vi "generate sensorion data log header.vi"(5 "line ending (\"\", none)":string, 7 "delimiter (comma)":string=", ", 9 "index format (-%02d)":string="%02d", 10 "num sensors":i32, 11 "header format (%15s)":string="%15s") -> (1 "delimiter":string, 2 "sensor data header string":string, 3 "value format":string)   [LabVIEW 2021]
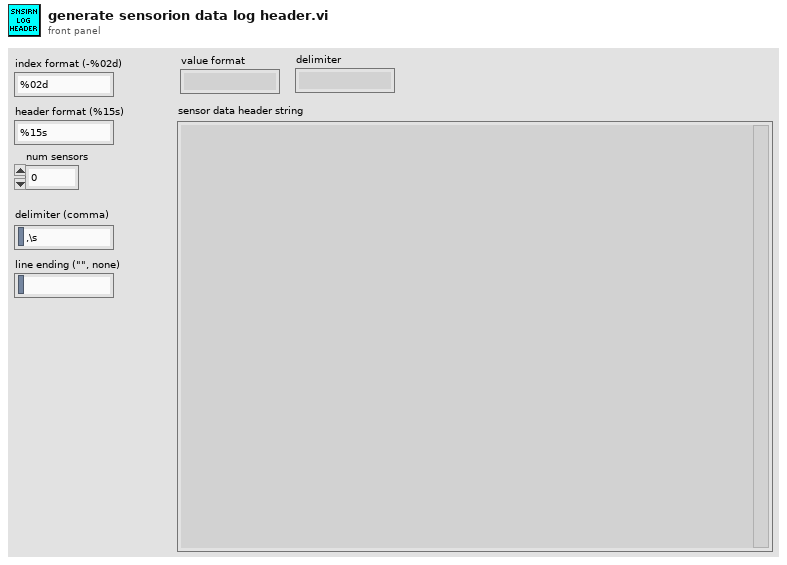
[diagram p1: front panel]
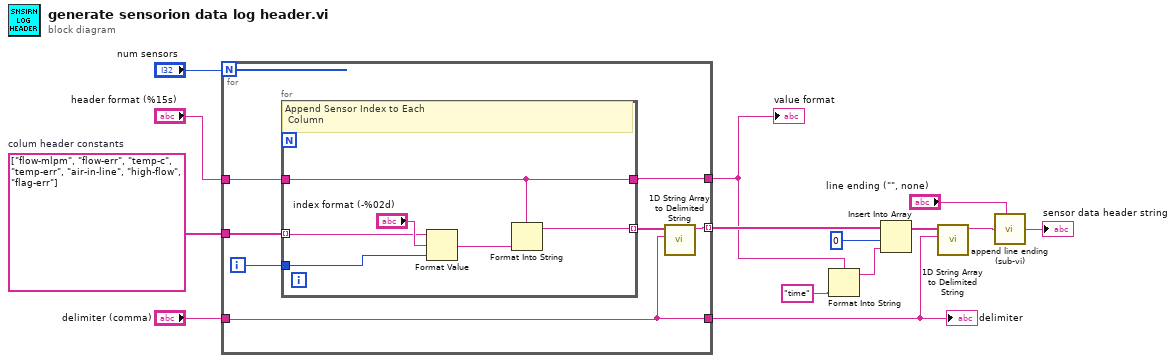
[diagram p0: block diagram]
diagram:
  w13 = string[] ["flow-mlpm", "flow-err", "temp-c", "temp-err", "air-in-line", "high-flow", "flag-err"]  # colum header constants
  n1 = for {
    N: "num sensors" -> [_]
    tunnel: w13 -> [w21]
    tunnel: "delimiter (comma)" -> [w18]
    tunnel: [w19] -> w9 mode=indexing
    tunnel: [w18] -> w11
    tunnel: "header format (%15s)" -> [w16]
    tunnel: [w15] -> w1
    i -> [w17]
    n2 = for {
      tunnel: w21 -> [w25] mode=indexing
      tunnel: w17 -> [w26]
      tunnel: [w23] -> w20 mode=indexing
      tunnel: w16 -> [w22]
      tunnel: [w22] -> w15
      # "Append Sensor Index to Each\n Column"
      n3 = Format Value(string ("")=w25, format string="index format (-%02d)", value (0)=w26) -> (output string=w24:string)
      n4 = Format Into String(format string=w22, w24) -> (resulting string=w23:string)  [unwired: 2 in, 1 out]
    }
    n5 = call <vilib>:"1D String Array to Delimited String.vi"("delimiter"=w18, "string array"=w20) -> ("delimited string"=w19:string)  [unwired: 9 in]
  }
  "value format" <- w1
  "delimiter" <- w11
  n6 = Format Into String(format string=w1, "time" ("new element/subarray")) -> (resulting string=w3:string)  [unwired: 2 in, 1 out]
  n7 = Insert Into Array(array=w9, index=0, new element=w3) -> (w10:string[])
  n8 = call <vilib>:"1D String Array to Delimited String.vi"("delimiter"=w11, "string array"=w10) -> ("delimited string"=w8:string)  [unwired: 9 in]
  n9 = call "append line ending (sub-vi).vi"("line ending (\\r\\n)"="line ending (\"\", none)", "string in"=w8) -> ("string out"=→"sensor data header string":string)  [unwired: 7 in]
